vi "RL-measurements.vi"(4 "WL final":dbl, 6 "WL initial":dbl, 7 "error in":errorcluster, 9 "RL Spectrum":dbl[](array[numeric]), 10 "WL Values":dbl[](array[numeric])) -> (0 "error out":errorcluster, 1 "FWHM":dbl, 2 "Peak value":dbl, 3 "Integration result":dbl, 5 "Peak WL":dbl)   [LabVIEW 2021]
doc: "Random Laser Project v2.0\nAndré Romero - 2024\nandretec@ifsc.usp.br"
uses:
  <vilib>/Analysis/2dsp.llb/Integral Method.ctl
  <vilib>/Analysis/8numeric.llb/1D Numeric Integration.vi
  <vilib>/Analysis/NI_AALPro.lvlib
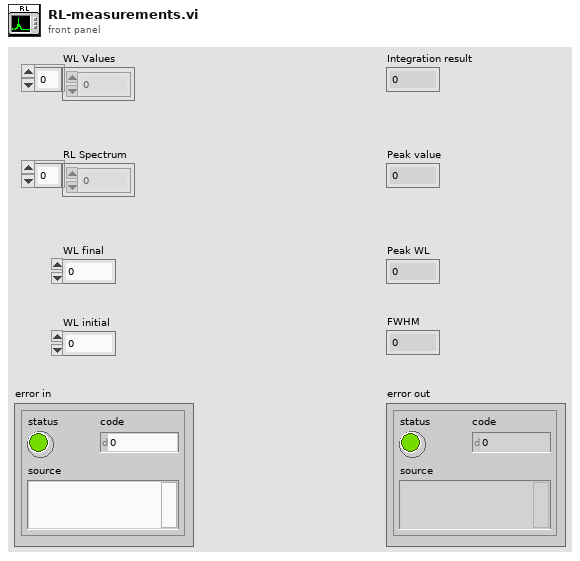
[diagram p1: front panel]
types:
  T1 = typedef "NI_AALPro.lvlib/Integral Method.ctl" = i32
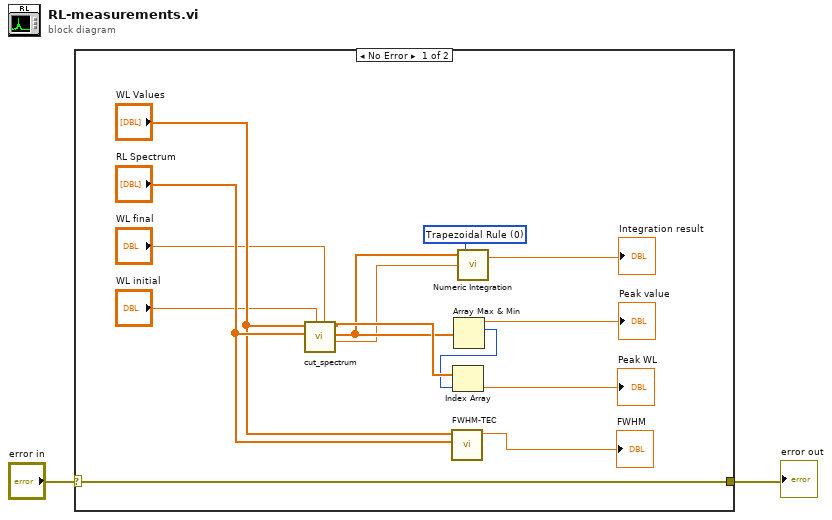
[diagram p0: block diagram]
diagram:
  n1 = case shown="No Error" "error in" {
    selector: "error in" -> [w3 w17]
    tunnel: [w3 w17] -> w1
    frame No Error {
      w7 = T1 0 items=["Trapezoidal Rule", "Simpson's Rule", "Simpson's 3/8 Rule", "Bode Rule"] ("integration method")
      n2 = call "cut_spectrum.vi"("WL Final"="WL final", "WL Initial"="WL initial", "RL Spectrum"="RL Spectrum", "WL Values"="WL Values") -> ("delta X"=w6:dbl, "RL Spectrum"=w15:dbl[], "WL Values"=w16:dbl[])  [unwired: 4 in, 1 out]
      n3 = call "FWHM-TEC.vi"("Y values"="RL Spectrum", "WL values"="WL Values") -> ("FWHM"=→"FWHM":dbl)  [unwired: 9 in]
      n4 = Array Max & Min(array=w15) -> (max value=→"Peak value":dbl, max index (indices)=w10:i32)  [unwired: 2 out]
      n5 = Index Array(array=w16, index=w10) -> (element=→"Peak WL":dbl)
      n6 = call-poly <vilib>:"Numeric Integration.vi"("integration method"=w7, "dt"=w6, "Input Array"=w15) -> ("result"=→"Integration result":dbl)  [unwired: 1 out]
    }
    frame Error {
    }
  }
  "error out" <- w1
